vi "UHR-Fleezers Control (host) - 12.1_Jonathan.vi"() -> ()   [LabVIEW 2012] (continued)
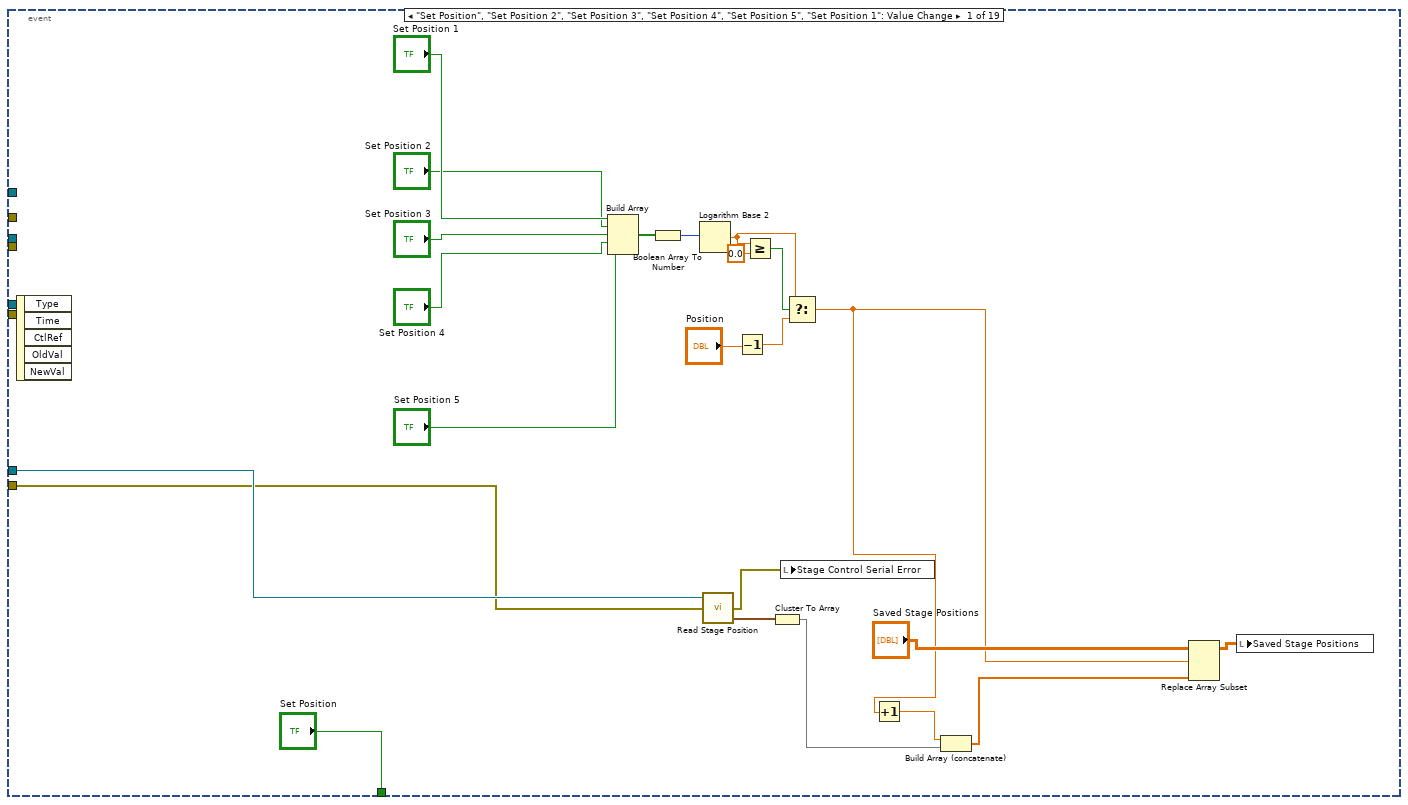
[diagram p3: hidden frame]
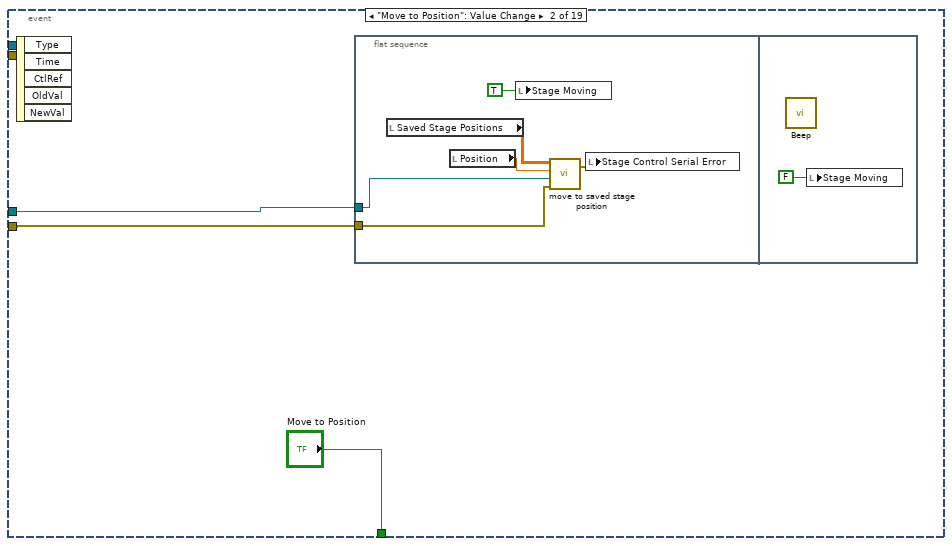
[diagram p4: hidden frame]
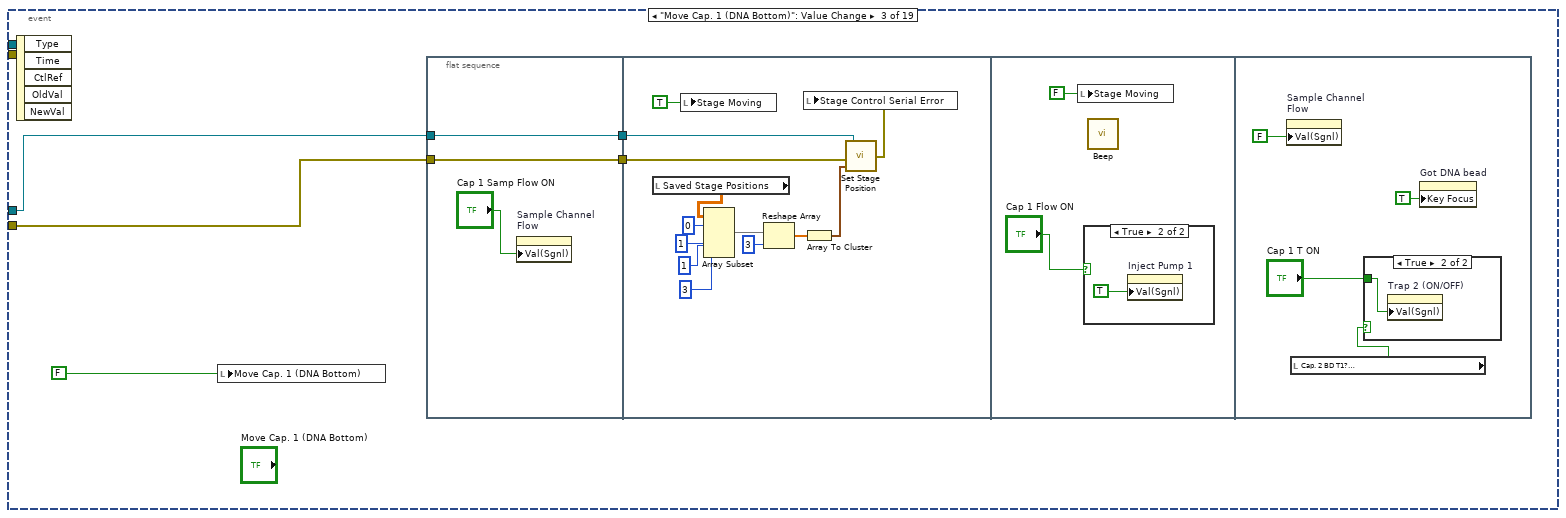
[diagram p5: hidden frame]
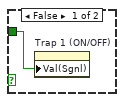
[diagram p7: hidden frame]
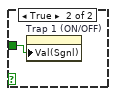
[diagram p9: hidden frame]
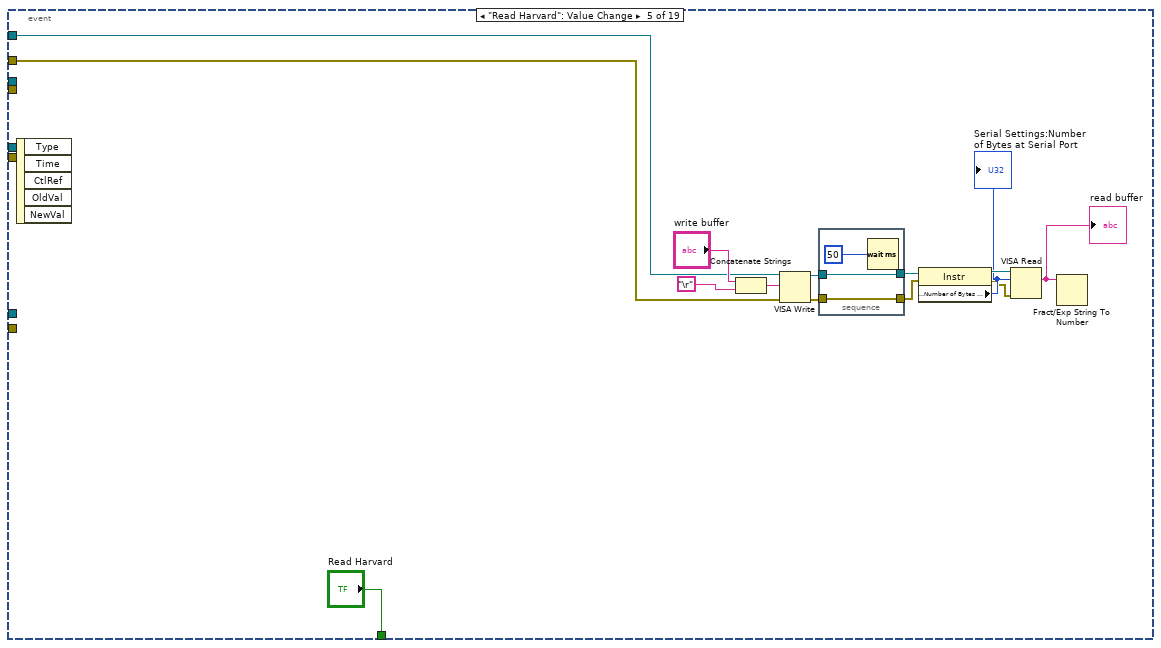
[diagram p10: hidden frame]
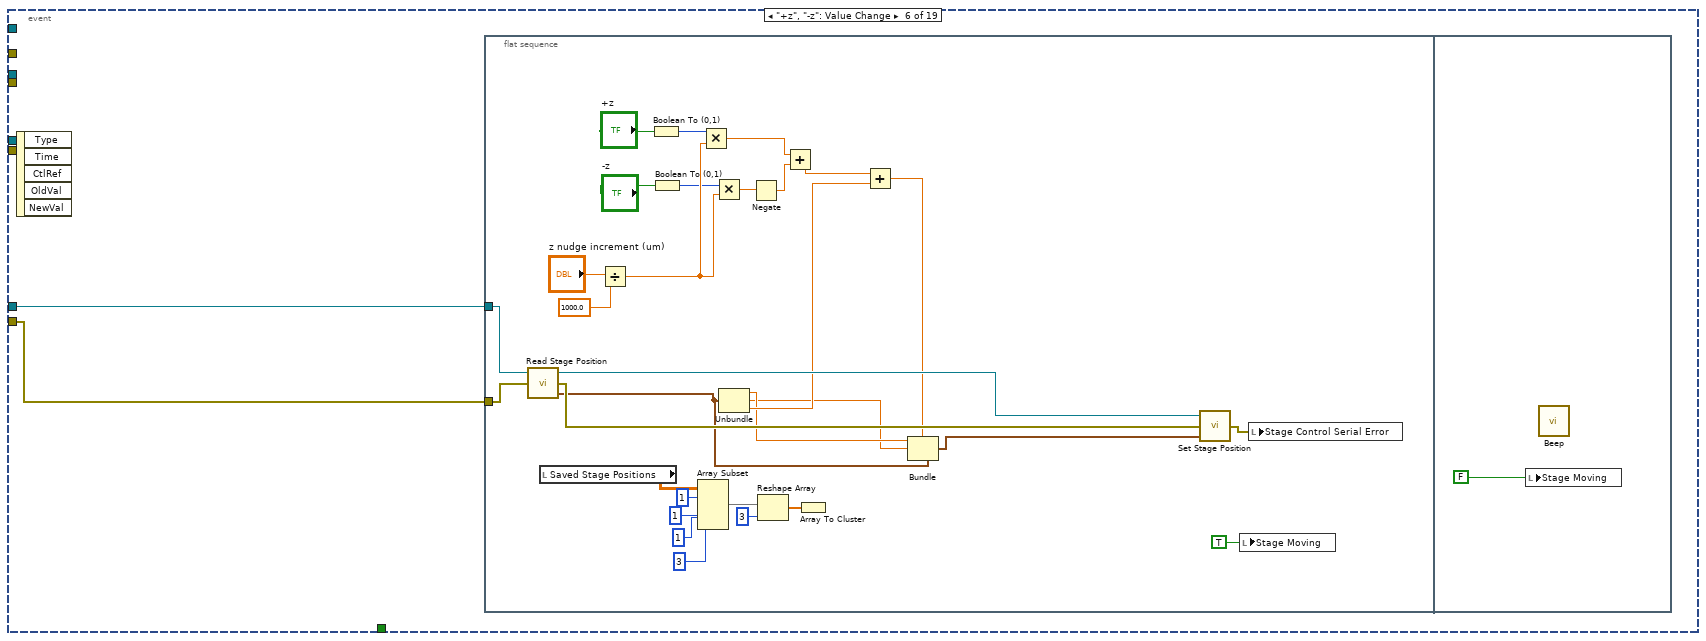
[diagram p11: hidden frame]
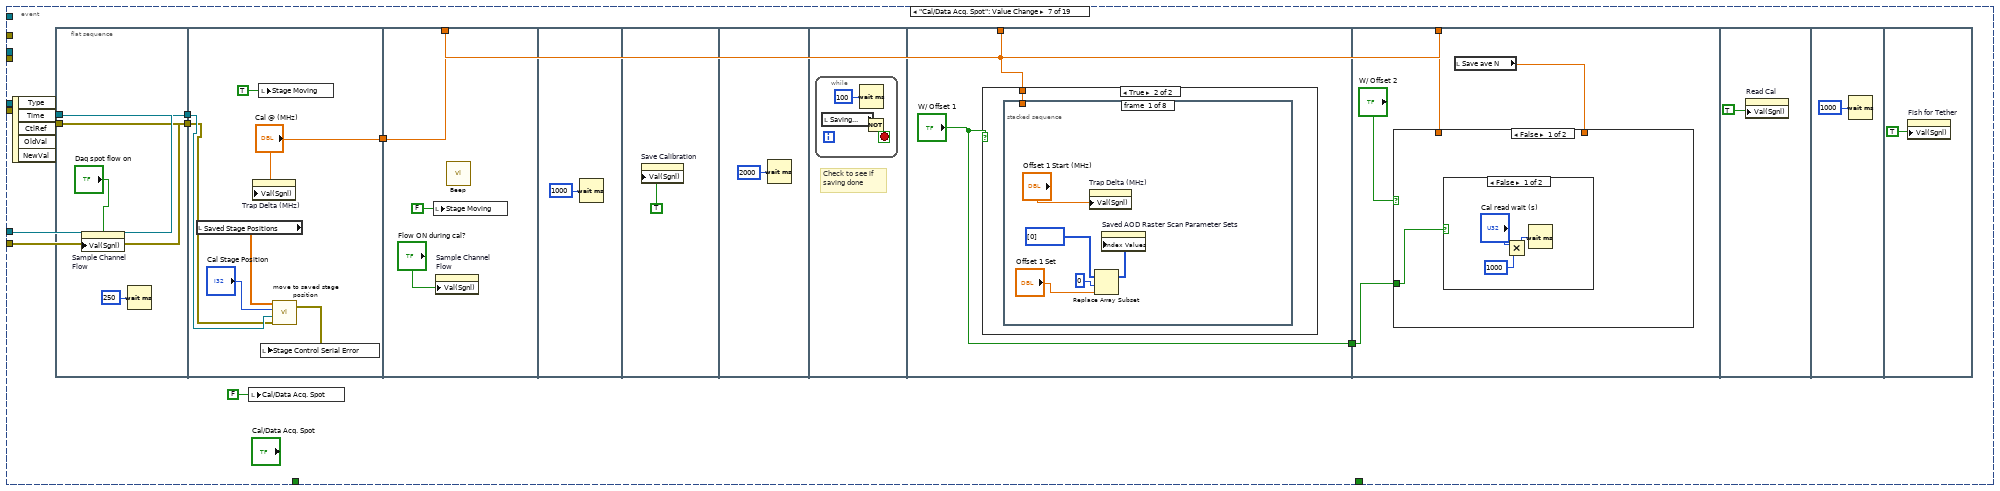
[diagram p12: hidden frame]
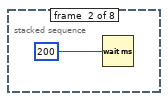
[diagram p14: hidden frame]
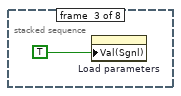
[diagram p15: hidden frame]
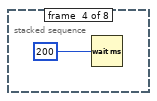
[diagram p16: hidden frame]
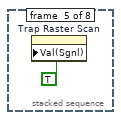
[diagram p17: hidden frame]
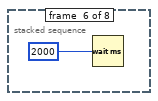
[diagram p18: hidden frame]
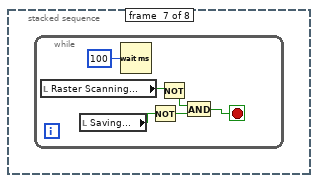
[diagram p19: hidden frame]
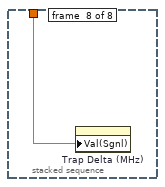
[diagram p20: hidden frame]
                                n2880 = property on="Rem fb disp offset" class="Bool (strict)"("Val(Sgnl)"=TRUE ("Value (Signaling)")) -> ()  [unwired: 2 in, 2 out]
                                }
                                }
                                }
                                frame True {
                                n2881 = flat-sequence {
                                tunnel: w4662 -> [w4663]
                                frame #0 {
                                n2882 = property on="Trap Delta (MHz)" class="DigNum (strict)"("Val(Sgnl)"=w4663) -> ()  [unwired: 2 in, 2 out]
                                }
                                frame #1 {
                                n2883 = Wait (ms)(milliseconds to wait=u32 500) -> ()  [unwired: 1 out]
                                }
                                frame #2 {
                                n2884 = local read "Shift confocal"() -> (w4669:bool)
                                n2885 = local read "Mean"() -> (w4670:dbl)
                                n2886 = Greater?(x=w4670, y=11.0) -> (0:w4668:bool)
                                n2887 = And(x=w4668, y=w4669) -> (x .and. y?=w4666:bool)
                                n2888 = Not(x=w4668) -> (.not. x?=w4667:bool)
                                n2889 = And(x=w4667, y=w4669) -> (x .and. y?=w4665:bool)
                                n2890 = case shown="True" w4666 {
                                frame False {
                                }
                                frame True {
                                n2891 = local read "Confocal Y 2 (V)"() -> (w4675:dbl)
                                n2892 = local read "Confocal X 2 (V)"() -> (w4674:dbl)
                                n2893 = property on="AO1" class="Slide (strict)"("Val(Sgnl)"=w4675) -> ()  [unwired: 2 in, 2 out]
                                n2894 = property on="AO2" class="Slide (strict)"("Val(Sgnl)"=w4674) -> ()  [unwired: 2 in, 2 out]
                                }
                                }
                                n2895 = case shown="True" w4665 {
                                frame False {
                                }
                                frame True {
                                n2896 = local read "Confocal Y 1 (V)"() -> (w4673:dbl)
                                n2897 = local read "Confocal X 1 (V)"() -> (w4672:dbl)
                                n2898 = property on="AO2" class="Slide (strict)"("Val(Sgnl)"=w4672) -> ()  [unwired: 2 in, 2 out]
                                n2899 = property on="AO1" class="Slide (strict)"("Val(Sgnl)"=w4673) -> ()  [unwired: 2 in, 2 out]
                                }
                                }
                                }
                                }
                                }
                                }
                                }
                                }
                                }
                                }
                                n2900 = local read "Time (s)"() -> (w4610:dbl)
                                n2901 = Subtract(x=w4611, y=w4610) -> (x-y=w4622:dbl)
                                n2902 = Number To Decimal String(number=w4622, width (-)=i16 0) -> (decimal integer string=w4620:string)
                                n2903 = Concatenate Strings(w4620, " s fluorescence event") -> (w4617:string)
                                n2904 = local read "Messages"() -> (w4618:string)
                                n2905 = local write "Duration (s)"(w4622) -> ()
                                n2906 = call "Update messages.vi"("Message to add"=w4617, "Old message string"=w4618) -> ("New message string"=w4616:string)
                                n2907 = local write "Messages"(w4616) -> ()
                                n2908 = call <vilib>:"Beep.vi"() -> ()  [unwired: 12 in]
                                n2909 = local write "Reset Force"(FALSE ("Force Reset")) -> ()
                                n2910 = local write "Fl. High"(TRUE ("Fl. High")) -> ()
                                n2911 = local write "Waiting"(TRUE ("Waiting")) -> ()
                                }
                                }
                                n2912 = node-c288() -> ()  [unwired: 1 in, 1 out]
                                }
                                n2913 = node-c288(w4589) -> ()  [unwired: 1 out]
                                }
                              }
                            }
                          }
                          n2914 = local read "Trap Delta (MHz)"() -> (w4501:dbl)
                          n2915 = local read "Trap Pos FB SP"() -> (w4499:fxp<+/-,16,1>)
                        }
                      }
                    }
                    frame True {
                      n2916 = flat-sequence {
                        tunnel: w4686 -> [w4696]
                        tunnel: [w4696] -> w4690
                        tunnel: w4689 -> [w4695]
                        tunnel: [w4695] -> w4688
                        tunnel: [w4694] -> w4687
                        tunnel: w4685 -> [w4693]
                        tunnel: [w4692] -> w4684
                        tunnel: w4681 -> [w4691]
                        tunnel: [w4691] -> w4680
                        tunnel: w4690 -> [w4766]
                        tunnel: w4688 -> [w4765]
                        tunnel: w4687 -> [w4764]
                        tunnel: w4684 -> [w4763]
                        tunnel: w4680 -> [w4762]
                        tunnel: [w4763] -> w4683
                        frame #0 {
                          n2917 = call <vilib>:"Beep.vi"() -> ()  [unwired: 3 in, 9 out]
                          n2918 = local write "Waiting"(FALSE ("Waiting")) -> ()
                          n2919 = Increment(x=w4693) -> (x+1=w4692:u8)
                          n2920 = case shown="\"Yank\"" w4695 {
                            tunnel: w4692 -> [_ _ w4702]
                            frame "Image" {
                              n2921 = property on="Confocal Image" class="Bool (strict)"("Val(Sgnl)"=TRUE ("Value (Signaling)")) -> ()  [unwired: 2 in, 2 out]
                            }
                            frame "Alarm", Default {
                            }
                            frame "Yank" {
                              n2922 = flat-sequence {
                                tunnel: w4702 -> [w4705]
                                tunnel: [w4704] -> w4701
                                tunnel: ["N Array El"] -> w4700
                                tunnel: w4701 -> [w4719]
                                tunnel: w4700 -> [w4715]
                                frame #0 {
                                n2923 = Multiply(x="Yank Delay (s)", y=1000.0) -> (x*y=w4708:dbl)
                                n2924 = Quotient & Remainder(x=w4705, y="N Array El") -> (x-y*floor(x/y)=w4704:u8)  [unwired: 1 out]
                                n2925 = Wait (ms)(milliseconds to wait=w4708) -> ()  [unwired: 1 out]
                                }
                                frame #1 {
                                n2926 = Random Number (0-1)() -> (number: 0 to 1=w4716:dbl)
                                n2927 = Multiply(x=w4715, y=w4716) -> (x*y=w4714:dbl)
                                n2928 = Round Toward -Infinity(1:w4714) -> (0:w4713:dbl)
                                n2929 = Select(t=w4713, s="Random Choice", f=w4719) -> (s? t:f=w4717:dbl)
                                n2930 = Select(t="Yank to Trap Delta (MHz)", s="Yank to which?", f="Yank to SP") -> (s? t:f=w4710:dbl[])
                                n2931 = Index Array(array=w4710, index=w4717) -> (element=w4720:dbl)
                                n2932 = case shown="False" "Yank to which?" {
                                tunnel: w4720 -> [w4721 w4747]
                                frame False {
                                n2933 = flat-sequence {
                                tunnel: w4721 -> [w4722]
                                frame #0 {
                                n2934 = property on="Trap Pos FB SP" class="DigNum (strict)"("Val(Sgnl)"=w4722) -> ()  [unwired: 2 in, 2 out]
                                }
                                frame #1 {
                                n2935 = Wait (ms)(milliseconds to wait=u32 700) -> ()  [unwired: 1 out]
                                }
                                frame #2 {
                                n2936 = local read "Action (%)"() -> (w4727:dbl)
                                n2937 = Absolute Value(x=w4727) -> (abs(x)=w4726:dbl)
                                n2938 = Greater?(x=w4726, y=70.0) -> (0:w4724:bool)
                                n2939 = property on="Remove Action Offset" class="Bool (strict)"("Val(Sgnl)"=w4724) -> ()  [unwired: 2 in, 2 out]
                                }
                                frame #3 {
                                n2940 = for {
                                N: 4 -> [_]
                                n2941 = flat-sequence {
                                frame #0 {
                                n2942 = Wait (ms)(milliseconds to wait=u32 500) -> ()  [unwired: 1 out]
                                }
                                frame #1 {
                                n2943 = local read "Action (%)"() -> (w4733:dbl)
                                n2944 = Absolute Value(x=w4733) -> (abs(x)=w4732:dbl)
                                n2945 = Greater?(x=w4732, y=70.0) -> (0:w4730:bool)
                                n2946 = property on="Remove Action Offset" class="Bool (strict)"("Val(Sgnl)"=w4730) -> ()  [unwired: 2 in, 2 out]
                                }
                                }
                                }
                                }
                                frame #4 {
                                n2947 = local read "Shift confocal"() -> (w4737:bool)
                                n2948 = local read "Mean"() -> (w4740:dbl)
                                n2949 = Greater?(x=w4740, y=11.0) -> (0:w4736:bool)
                                n2950 = Not(x=w4736) -> (.not. x?=w4735:bool)
                                n2951 = And(x=w4735, y=w4737) -> (x .and. y?=w4734:bool)
                                n2952 = And(x=w4736, y=w4737) -> (x .and. y?=w4738:bool)
                                n2953 = case shown="True" w4738 {
                                frame False {
                                }
                                frame True {
                                n2954 = local read "Confocal X 2 (V)"() -> (w4743:dbl)
                                n2955 = local read "Confocal Y 2 (V)"() -> (w4744:dbl)
                                n2956 = property on="AO2" class="Slide (strict)"("Val(Sgnl)"=w4743) -> ()  [unwired: 2 in, 2 out]
                                n2957 = property on="AO1" class="Slide (strict)"("Val(Sgnl)"=w4744) -> ()  [unwired: 2 in, 2 out]
                                }
                                }
                                n2958 = case shown="True" w4734 {
                                frame False {
                                }
                                frame True {
                                n2959 = local read "Confocal X 1 (V)"() -> (w4741:dbl)
                                n2960 = local read "Confocal Y 1 (V)"() -> (w4742:dbl)
                                n2961 = property on="AO1" class="Slide (strict)"("Val(Sgnl)"=w4742) -> ()  [unwired: 2 in, 2 out]
                                n2962 = property on="AO2" class="Slide (strict)"("Val(Sgnl)"=w4741) -> ()  [unwired: 2 in, 2 out]
                                }
                                }
                                }
                                frame #5 {
                                n2963 = Wait (ms)(milliseconds to wait=u32 1500) -> ()  [unwired: 1 out]
                                }
                                frame #6 {
                                n2964 = property on="Rem fb disp offset" class="Bool (strict)"("Val(Sgnl)"=TRUE ("Value (Signaling)")) -> ()  [unwired: 2 in, 2 out]
                                }
                                }
                                }
                                frame True {
                                n2965 = flat-sequence {
                                tunnel: w4747 -> [w4748]
                                frame #0 {
                                n2966 = property on="Trap Delta (MHz)" class="DigNum (strict)"("Val(Sgnl)"=w4748) -> ()  [unwired: 2 in, 2 out]
                                }
                                frame #1 {
                                n2967 = Wait (ms)(milliseconds to wait=u32 500) -> ()  [unwired: 1 out]
                                }
                                frame #2 {
                                n2968 = local read "Shift confocal"() -> (w4752:bool)
                                n2969 = local read "Mean"() -> (w4750:dbl)
                                n2970 = Greater?(x=w4750, y=11.0) -> (0:w4753:bool)
                                n2971 = Not(x=w4753) -> (.not. x?=w4754:bool)
                                n2972 = And(x=w4754, y=w4752) -> (x .and. y?=w4756:bool)
                                n2973 = And(x=w4753, y=w4752) -> (x .and. y?=w4755:bool)
                                n2974 = case shown="True" w4755 {
                                frame False {
                                }
                                frame True {
                                n2975 = local read "Confocal Y 2 (V)"() -> (w4760:dbl)
                                n2976 = local read "Confocal X 2 (V)"() -> (w4759:dbl)
                                n2977 = property on="AO1" class="Slide (strict)"("Val(Sgnl)"=w4760) -> ()  [unwired: 2 in, 2 out]
                                n2978 = property on="AO2" class="Slide (strict)"("Val(Sgnl)"=w4759) -> ()  [unwired: 2 in, 2 out]
                                }
                                }
                                n2979 = case shown="True" w4756 {
                                frame False {
                                }
                                frame True {
                                n2980 = local read "Confocal X 1 (V)"() -> (w4757:dbl)
                                n2981 = local read "Confocal Y 1 (V)"() -> (w4758:dbl)
                                n2982 = property on="AO2" class="Slide (strict)"("Val(Sgnl)"=w4757) -> ()  [unwired: 2 in, 2 out]
                                n2983 = property on="AO1" class="Slide (strict)"("Val(Sgnl)"=w4758) -> ()  [unwired: 2 in, 2 out]
                                }
                                }
                                }
                                }
                                }
                                }
                                }
                              }
                            }
                          }
                          n2984 = local read "Time (s)"() -> (w4694:dbl)
                          "Fl. High" <- TRUE ("Yanking")
                        }
                        frame #1 {
                          n2985 = local read "Auto F Reset"() -> (w4761:bool)
                          n2986 = case shown="True" w4761 {
                            tunnel: w4766 -> [_ w4770]
                            tunnel: w4765 -> [_ w4769]
                            tunnel: w4764 -> [_ w4768]
                            tunnel: w4762 -> [_ w4767]
                            frame False {
                            }
                            frame True {
                              n2987 = node-c288() -> (w4772:T22)  [unwired: 4 out]
                              n2988 = timed-loop {
                                timing: w4772 -> [_]
                                timing-out: [_] -> w4771
                                tunnel: w4770 -> [w4790]
                                tunnel: w4769 -> [w4789]
                                tunnel: w4768 -> [w4788]
                                tunnel: w4767 -> [w4787]
                                stop <- w4773 stop-if-true
                                n2989 = node-c288() -> ()  [unwired: 2 out]
                                n2990 = local read "Fl. Delta Thresh. (kHz)"() -> (w4781:dbl)
                                n2991 = local read "Fl. Triggered..."() -> (w4786:bool)
                                n2992 = local read "Delta Fl. 1"() -> (w4777:dbl)
                                n2993 = local read "Delta Fl. 2"() -> (w4775:dbl)
                                n2994 = local read "Stop All"() -> (w4784:bool)
                                n2995 = local read "APD to Watch"() -> (w4776:bool)
                                n2996 = Select(t=w4777, s=w4776, f=w4775) -> (s? t:f=w4774:dbl)
                                n2997 = Not(x=w4786) -> (.not. x?=w4785:bool)
                                n2998 = Multiply(x=w4781, y=1000.0) -> (x*y=w4780:dbl)
                                n2999 = Negate(x=w4780) -> (-x=w4779:dbl)
                                n3000 = Less?(x=w4774, y=w4779) -> (x < y?=w4783:bool)
                                n3001 = Compound Arithmetic op=OR(w4783, w4784, w4785, "Reset Force") -> (w4773:bool)
                                n3002 = case shown="True" w4773 {
                                tunnel: w4790 -> [_ w4805]
                                tunnel: w4789 -> [_ w4804]
                                tunnel: w4788 -> [_ w4794]
                                tunnel: w4787 -> [_ w4796]
                                frame False {
                                }
                                frame True {
                                n3003 = local read "Time (s)"() -> (w4795:dbl)
                                n3004 = case shown="\"Yank\"" w4804 {
                                tunnel: w4805 -> [_ w4808]
                                tunnel: w4796 -> [_ w4806]
                                frame "Image", Default {
                                }
                                frame "Yank" {
                                n3005 = flat-sequence {
                                tunnel: [w4814] -> w4809
                                tunnel: w4808 -> [w4814]
                                tunnel: [w4810] -> w4807
                                tunnel: w4806 -> [w4810]
                                tunnel: w4809 -> [w4817]
                                tunnel: w4807 -> [w4815]
                                frame #0 {
                                n3006 = local read "Yank Delay (s)"() -> (w4813:dbl)
                                n3007 = Multiply(x=w4813, y=1000.0) -> (x*y=w4811:dbl)
                                n3008 = Wait (ms)(milliseconds to wait=w4811) -> ()  [unwired: 1 out]
                                }
                                frame #1 {
                                n3009 = local read "Yank to which?"() -> (w4816:bool)
                                n3010 = case shown="False" w4816 {
                                tunnel: w4817 -> [_ w4844]
                                tunnel: w4815 -> [w4818 _]
                                frame False {
                                n3011 = flat-sequence {
                                tunnel: w4818 -> [w4819]
                                frame #0 {
                                n3012 = property on="Trap Pos FB SP" class="DigNum (strict)"("Val(Sgnl)"=w4819) -> ()  [unwired: 2 in, 2 out]
                                }
                                frame #1 {
                                n3013 = Wait (ms)(milliseconds to wait=u32 700) -> ()  [unwired: 1 out]
                                }
                                frame #2 {
                                n3014 = local read "Action (%)"() -> (w4824:dbl)
                                n3015 = Absolute Value(x=w4824) -> (abs(x)=w4823:dbl)
                                n3016 = Greater?(x=w4823, y=70.0) -> (0:w4821:bool)
                                n3017 = property on="Remove Action Offset" class="Bool (strict)"("Val(Sgnl)"=w4821) -> ()  [unwired: 2 in, 2 out]
                                }
                                frame #3 {
                                n3018 = for {
                                N: 4 -> [_]
                                n3019 = flat-sequence {
                                frame #0 {
                                n3020 = Wait (ms)(milliseconds to wait=u32 500) -> ()  [unwired: 1 out]
                                }
                                frame #1 {
                                n3021 = local read "Action (%)"() -> (w4830:dbl)
                                n3022 = Absolute Value(x=w4830) -> (abs(x)=w4829:dbl)
                                n3023 = Greater?(x=w4829, y=70.0) -> (0:w4827:bool)
                                n3024 = property on="Remove Action Offset" class="Bool (strict)"("Val(Sgnl)"=w4827) -> ()  [unwired: 2 in, 2 out]
                                }
                                }
                                }
                                }
                                frame #4 {
                                n3025 = local read "Shift confocal"() -> (w4835:bool)
                                n3026 = local read "Mean"() -> (w4837:dbl)
                                n3027 = Greater?(x=w4837, y=11.0) -> (0:w4834:bool)
                                n3028 = Not(x=w4834) -> (.not. x?=w4833:bool)
                                n3029 = And(x=w4834, y=w4835) -> (x .and. y?=w4832:bool)
                                n3030 = And(x=w4833, y=w4835) -> (x .and. y?=w4831:bool)
                                n3031 = case shown="True" w4832 {
                                frame False {
                                }
                                frame True {
                                n3032 = local read "Confocal Y 2 (V)"() -> (w4841:dbl)
                                n3033 = local read "Confocal X 2 (V)"() -> (w4840:dbl)
                                n3034 = property on="AO2" class="Slide (strict)"("Val(Sgnl)"=w4840) -> ()  [unwired: 2 in, 2 out]
                                n3035 = property on="AO1" class="Slide (strict)"("Val(Sgnl)"=w4841) -> ()  [unwired: 2 in, 2 out]
                                }
                                }
                                n3036 = case shown="True" w4831 {
                                frame False {
                                }
                                frame True {
                                n3037 = local read "Confocal X 1 (V)"() -> (w4838:dbl)
                                n3038 = local read "Confocal Y 1 (V)"() -> (w4839:dbl)
                                n3039 = property on="AO1" class="Slide (strict)"("Val(Sgnl)"=w4839) -> ()  [unwired: 2 in, 2 out]
                                n3040 = property on="AO2" class="Slide (strict)"("Val(Sgnl)"=w4838) -> ()  [unwired: 2 in, 2 out]
                                }
                                }
                                }
                                frame #5 {
                                n3041 = Wait (ms)(milliseconds to wait=u32 1500) -> ()  [unwired: 1 out]
                                }
                                frame #6 {
                                n3042 = property on="Rem fb disp offset" class="Bool (strict)"("Val(Sgnl)"=TRUE ("Value (Signaling)")) -> ()  [unwired: 2 in, 2 out]
                                }
                                }
                                }
                                frame True {
                                n3043 = flat-sequence {
                                tunnel: w4844 -> [w4845]
                                frame #0 {
                                n3044 = property on="Trap Delta (MHz)" class="DigNum (strict)"("Val(Sgnl)"=w4845) -> ()  [unwired: 2 in, 2 out]
                                }
                                frame #1 {
                                n3045 = Wait (ms)(milliseconds to wait=u32 500) -> ()  [unwired: 1 out]
                                }
                                frame #2 {
                                n3046 = local read "Shift confocal"() -> (w4851:bool)
                                n3047 = local read "Mean"() -> (w4853:dbl)
                                n3048 = Greater?(x=w4853, y=11.0) -> (0:w4850:bool)
                                n3049 = Not(x=w4850) -> (.not. x?=w4849:bool)
                                n3050 = And(x=w4850, y=w4851) -> (x .and. y?=w4848:bool)
                                n3051 = And(x=w4849, y=w4851) -> (x .and. y?=w4847:bool)
                                n3052 = case shown="True" w4848 {
                                frame False {
                                }
                                frame True {
                                n3053 = local read "Confocal Y 2 (V)"() -> (w4857:dbl)
                                n3054 = local read "Confocal X 2 (V)"() -> (w4856:dbl)
                                n3055 = property on="AO2" class="Slide (strict)"("Val(Sgnl)"=w4856) -> ()  [unwired: 2 in, 2 out]
                                n3056 = property on="AO1" class="Slide (strict)"("Val(Sgnl)"=w4857) -> ()  [unwired: 2 in, 2 out]
                                }
                                }
                                n3057 = case shown="True" w4847 {
                                frame False {
                                }
                                frame True {
                                n3058 = local read "Confocal Y 1 (V)"() -> (w4855:dbl)
                                n3059 = local read "Confocal X 1 (V)"() -> (w4854:dbl)
                                n3060 = property on="AO2" class="Slide (strict)"("Val(Sgnl)"=w4854) -> ()  [unwired: 2 in, 2 out]
                                n3061 = property on="AO1" class="Slide (strict)"("Val(Sgnl)"=w4855) -> ()  [unwired: 2 in, 2 out]
                                }
                                }
                                }
                                }
                                }
                                }
                                }
                                }
                                }
                                }
                                n3062 = local read "Messages"() -> (w4803:string)
                                n3063 = Subtract(x=w4795, y=w4794) -> (x-y=w4801:dbl)
                                "Duration (s)" <- w4801
                                n3064 = Number To Decimal String(number=w4801, width (-)=i16 0) -> (decimal integer string=w4799:string)
                                n3065 = Concatenate Strings(w4799, " s fluorescence event." ("string")) -> (w4797:string)
                                n3066 = call "Update messages.vi"("Message to add"=w4797, "Old message string"=w4803) -> ("New message string"=w4802:string)
                                n3067 = local write "Reset Force"(FALSE ("Reset Force")) -> ()
                                n3068 = local write "Waiting"(TRUE ("Waiting")) -> ()
                                n3069 = local write "Messages"(w4802) -> ()
                                n3070 = local write "Fl. High"(FALSE ("Fl. High")) -> ()
                                n3071 = call <vilib>:"Beep.vi"() -> ()  [unwired: 3 in, 9 out]
                                }
                                }
                                n3072 = node-c288() -> ()  [unwired: 2 out]
                              }
                              n3073 = node-c288(w4771) -> ()  [unwired: 1 out]
                            }
                          }
                        }
                      }
                      n3074 = local read "Trap Delta (MHz)"() -> (w4686:dbl)
                      n3075 = local read "Trap Pos FB SP"() -> (w4681:fxp<+/-,16,1>)
                    }
                  }
                }
                frame #1 {
                  n3076 = local read "Stop All"() -> (w4867:bool)
                  n3077 = local read "Fl. Triggered..."() -> (w4865:bool)
                  n3078 = Not(x=w4865) -> (.not. x?=w4866:bool)
                  n3079 = Or(x=w4866, y=w4867) -> (x .or. y?=w4864:bool)
                }
              }
              n3080 = case shown="True" w4458 {
                frame False {
                }
                frame True {
                  n3081 = local read "Confocal Y 1 (V)"() -> (w4468:dbl)
                  n3082 = local read "Confocal X 1 (V)"() -> (w4467:dbl)
                  n3083 = property on="AO2" class="Slide (strict)"("Val(Sgnl)"=w4467) -> ()  [unwired: 2 in, 2 out]
                  n3084 = property on="AO1" class="Slide (strict)"("Val(Sgnl)"=w4468) -> ()  [unwired: 2 in, 2 out]
                }
              }
              n3085 = case shown="True" w4458 {
                frame False {
                }
                frame True {
                  w4466 = FALSE ("Fl. High")
                  n3086 = local write "Waiting"(w4466) -> ()
                  n3087 = local write "Fl. High"(w4466) -> ()
                }
              }
              n3088 = node-c288() -> ()  [unwired: 2 out]
            }
            n3089 = node-c288(w4456) -> ()  [unwired: 1 out]
          }
        }
      }
      event "Stop All": Value Change {
        n3090 = event-data() -> ()  [unwired: 7 out]
        n3091 = local read "Stop All"() -> (w4872:bool)
      }
    }
    n3092 = node-c288() -> ()  [unwired: 2 out]
  }
  n3093 = node-c288(w98) -> ()  [unwired: 1 out]
  n3094 = node-c288(w100) -> ()  [unwired: 1 out]
  n3095 = node-c288(w85) -> ()  [unwired: 1 out]
  n3096 = property on="Saved trap pos" class="WFGraph (strict)"("Visible"=FALSE) -> ()  [unwired: 2 in, 2 out]
  n3097 = property on="Trap Delta Graph" class="WFGraph (strict)"("Visible"=TRUE) -> ()  [unwired: 2 in, 2 out]
  n3098 = local write "Trap pos"(FALSE ("Trap pos")) -> ()
  n3099 = local write "Offset (nm)"(0.0 ("Offset (nm)")) -> ()
  n3100 = local write "Bead Mean (nm)"(0.0 ("Bead Mean (nm)")) -> ()
  n3101 = disable-structure shown="Disabled" {
    disable-tunnel: w89 -> [w4874 _]
    disable-tunnel: w88 -> [w4873 _]
    frame Disabled {
      n3102 = VISA Close(VISA resource name=w4874, error in (no error)=w4873) -> (error out=w4875:errorcluster)
      n3103 = call <vilib>:"Simple Error Handler.vi"("error in (no error)"=w4875) -> ()  [unwired: 1 in, 8 out]
    }
    frame Enabled {
    }
  }
  n3104 = node-c288(w180) -> ()  [unwired: 1 out]
  n3105 = node-c288(w96) -> ()  [unwired: 1 out]
  n3106 = flat-sequence {
    tunnel: w274 -> [w4879]
    tunnel: w276 -> [w4880]
    tunnel: [w4878] -> w255
    tunnel: [w4877] -> w254
    tunnel: w236 -> [_]
    tunnel: w188 -> [_]
    tunnel: w102 -> [_]
    tunnel: w255 -> [w4881]
    tunnel: w254 -> [w4882]
    frame #0 {
      w4876 = FALSE ("AI to FIFO")
      n3107 = xnode "Read/Write Control"("FPGA VI Reference In"=w4880, "error in"=w4879, "AI to FIFO"=w4876, "APD to FIFO"=w4876) -> ("FPGA VI Reference Out"=w4878:T20, "error out"=w4877:errorcluster)
    }
    frame #1 {
      n3108 = xnode "Close FPGA VI Reference"("FPGA VI Reference In"=w4881, "error in"=w4882) -> ("error out"=→"error out":errorcluster)
    }
    frame #2 {
      n3109 = local read "connection reference"() -> (w4884:T1)
      n3110 = call <vilib>:"DB Tools Close Connection.vi"("connection reference"=w4884) -> ()  [unwired: 6 in, 1 out]
    }
  }
